vi "Servos.vi"(0 "Stop Button":bool, 1 "Servo DC":cluster{"1":u32, "2":u32, "3":u32, "4":u32}) -> ()   [LabVIEW 2015]
uses:
  <vilib>/rvi/Emulation/niFpgaGetClockAttributes.vi
  <vilib>/rvi/Emulation/niFpgaSctlEmulationGetInTimedLoop.vi
  <vilib>/rvi/Emulation/niFpgaEmulationReportErrorSimple.vi
  <vilib>/rvi/eio/common/nirviEmuTemplateMethod_errors.vi
  <vilib>/rvi/Emulation/niFpgaProcessEmulError.vi
  <vilib>/rvi/Emulation/niFpgaCriticalErrorInLSC.vi
  <vilib>/eio/EIONode/EIONode.xnode
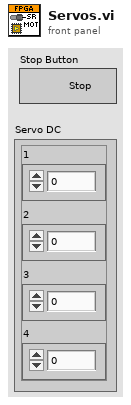
[diagram p1: front panel]
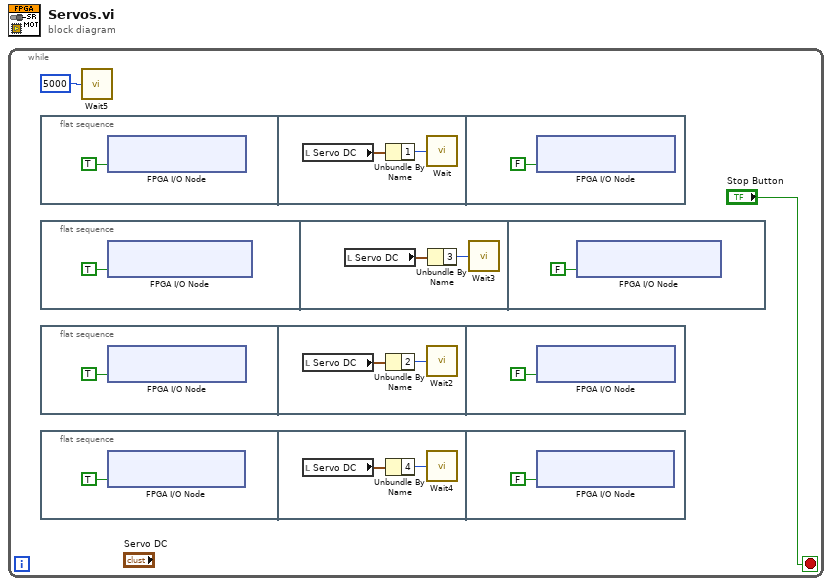
[diagram p0: block diagram]
diagram:
  n1 = while {
    stop <- "Stop Button" stop-if-true
    n2 = flat-sequence {
      frame #0 {
        n3 = xnode "FPGA I/O Node"("ConnectorA/DIO8"=TRUE) -> ()  [unwired: 1 in, 1 out]
      }
      frame #1 {
        n4 = local read "Servo DC"() -> (w5:cluster{"1":u32, "2":u32, "3":u32, "4":u32})
        n5 = Unbundle By Name(w5) -> ("1"=w4:u32)
        n6 = call "Wait"("Count(uSec)"=w4) -> ()  [unwired: 1 out]
      }
      frame #2 {
        n7 = xnode "FPGA I/O Node"("ConnectorA/DIO8"=FALSE) -> ()  [unwired: 1 in, 1 out]
      }
    }
    n8 = flat-sequence {
      frame #0 {
        n9 = xnode "FPGA I/O Node"("ConnectorA/DIO10"=TRUE) -> ()  [unwired: 1 in, 1 out]
      }
      frame #1 {
        n10 = local read "Servo DC"() -> (w9:cluster{"1":u32, "2":u32, "3":u32, "4":u32})
        n11 = Unbundle By Name(w9) -> ("3"=w8:u32)
        n12 = call "Wait3"("Count(uSec)"=w8) -> ()  [unwired: 1 out]
      }
      frame #2 {
        n13 = xnode "FPGA I/O Node"("ConnectorA/DIO10"=FALSE) -> ()  [unwired: 1 in, 1 out]
      }
    }
    n14 = flat-sequence {
      frame #0 {
        n15 = xnode "FPGA I/O Node"("ConnectorA/DIO9"=TRUE) -> ()  [unwired: 1 in, 1 out]
      }
      frame #1 {
        n16 = local read "Servo DC"() -> (w13:cluster{"1":u32, "2":u32, "3":u32, "4":u32})
        n17 = Unbundle By Name(w13) -> ("2"=w12:u32)
        n18 = call "Wait2"("Count(uSec)"=w12) -> ()  [unwired: 1 out]
      }
      frame #2 {
        n19 = xnode "FPGA I/O Node"("ConnectorA/DIO9"=FALSE) -> ()  [unwired: 1 in, 1 out]
      }
    }
    n20 = flat-sequence {
      frame #0 {
        n21 = xnode "FPGA I/O Node"("ConnectorB/DIO8"=TRUE) -> ()  [unwired: 1 in, 1 out]
      }
      frame #1 {
        n22 = local read "Servo DC"() -> (w17:cluster{"1":u32, "2":u32, "3":u32, "4":u32})
        n23 = Unbundle By Name(w17) -> ("4"=w16:u32)
        n24 = call "Wait4"("Count(uSec)"=w16) -> ()  [unwired: 1 out]
      }
      frame #2 {
        n25 = xnode "FPGA I/O Node"("ConnectorB/DIO8"=FALSE) -> ()  [unwired: 1 in, 1 out]
      }
    }
    n26 = call "Wait5"("Count(uSec)"=u32 5000) -> ()  [unwired: 1 out]
  }
